vi "simulaVolt.vi"(8 "error in (no error)":errorcluster, 10 "volt in":dbl=0.75 format="%#_13g") -> (0 "error out":errorcluster, 2 "volt out":dbl)   [LabVIEW 2019, in "K2002_GPIB.lvlib"]
uses:
  K2002_GPIB.lvlib
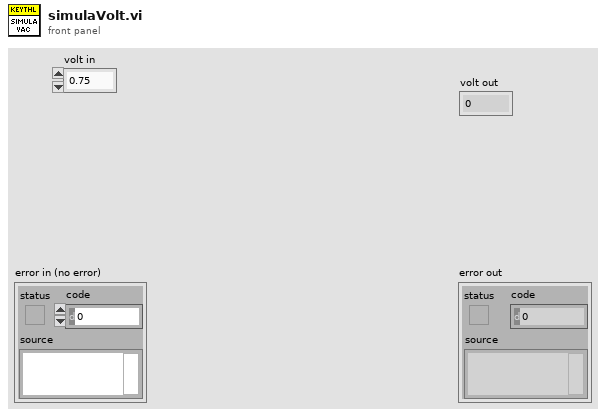
[diagram p1: front panel]
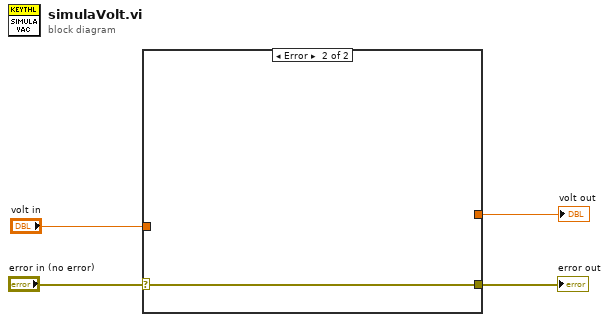
[diagram p0: block diagram]
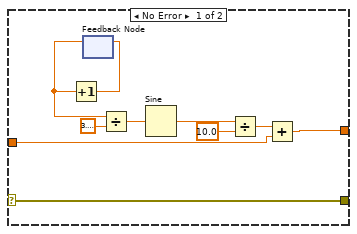
[diagram p2: hidden frame]
diagram:
  n1 = case shown="Error" "error in (no error)" {
    selector: "error in (no error)" -> [w14 w15]
    tunnel: [w14 w15] -> w3
    tunnel: "volt in" -> [w8 _]
    tunnel: [w7 _] -> w1
    frame No Error {
      n2 = feedback #1() -> (w9:dbl)  [unwired: 1 in]
      n3 = Increment(x=w9) -> (x+1=w13:dbl)
      n4 = feedback-in #1(w13) -> ()
      n5 = Divide(x=w9, y=3.141592653589793) -> (x/y=w12:dbl)
      n6 = Sine(x=w12) -> (sin(x)=w10:dbl)
      n7 = Divide(x=w10, y=10.0) -> (x/y=w6:dbl)
      n8 = Add(x=w6, y=w8) -> (x+y=w7:dbl)
    }
    frame Error {
    }
  }
  "error out" <- w3
  "volt out" <- w1
